vi "Clear Scan Time Out_2.vi"(6 "Channel number":i32, 7 "ESP32 ref":refnum<visa-resource-name>="COM4", 8 "error in (no error)":errorcluster, 11 "VISA Refnum in":refnum<visa-resource-name>) -> (0 "error out":errorcluster, 1 "error?":bool, 2 "Time out count":i32, 3 "VISA Refnum out":refnum<visa-resource-name>, 5 "ESP32 ref out":refnum<visa-resource-name>)   [LabVIEW 2023]
uses:
  <vilib>/Utility/error.llb/DialogType.ctl
panel:
  out "error out 3":errorcluster
  out "error out 2":errorcluster
  out "Measurements 3":dbl[](array[numeric])
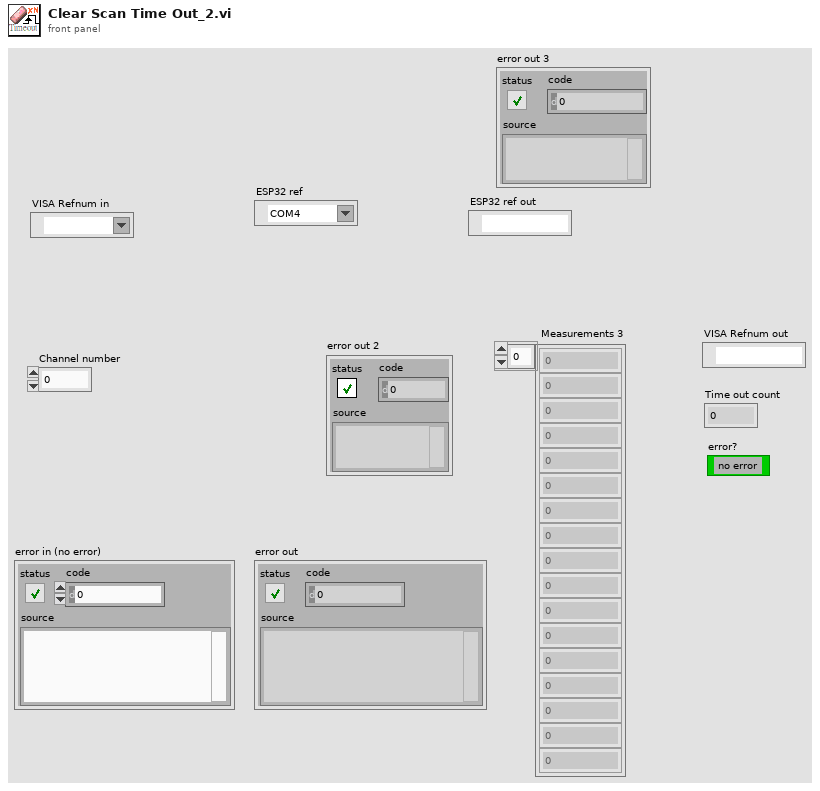
[diagram p1: front panel]
types:
  T1 = typedef "DialogType.ctl" = u16
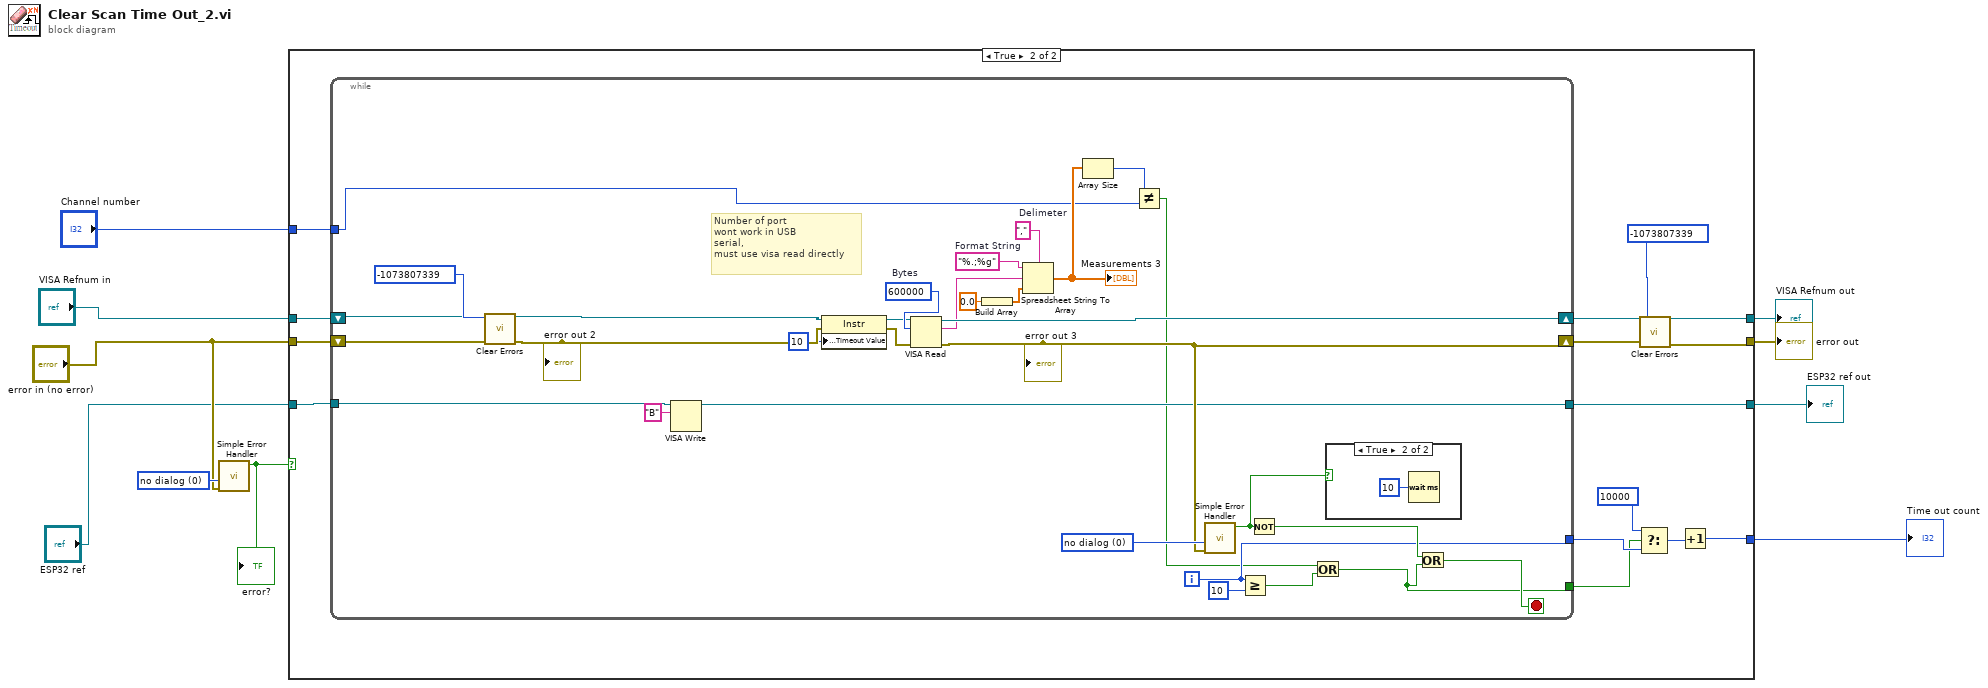
[diagram p0: block diagram]
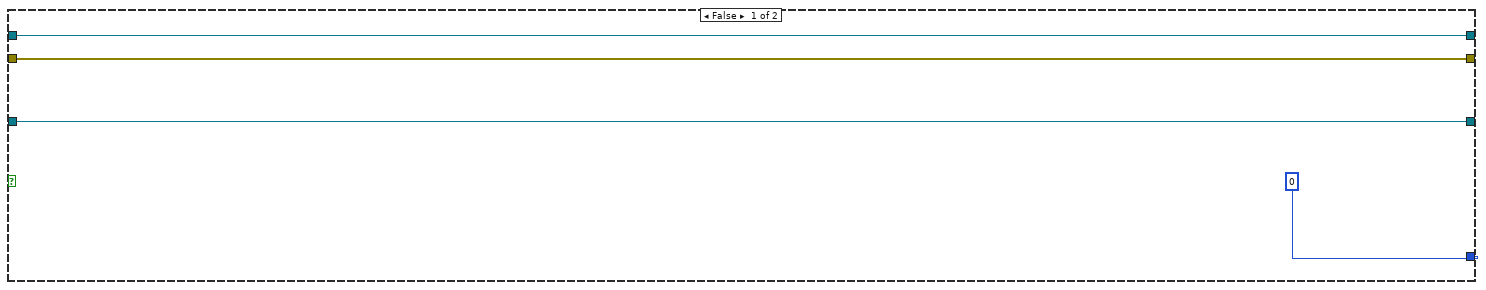
[diagram p2: hidden frame]
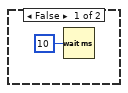
[diagram p3: hidden frame]
diagram:
  w7 = T1 0 items=["no dialog", "OK message", "continue or stop message", "OK message + warnings", "continue/stop + warnings"] ("type of dialog (OK msg:1)")
  n1 = call <vilib>:"Simple Error Handler.vi"("type of dialog (OK msg:1)"=w7, "error in (no error)"="error in (no error)") -> ("error?"=w5:bool)  [unwired: 3 in, 4 out]
  "error?" <- w5
  n2 = case shown="True" w5 {
    tunnel: [w14 w28] -> w10
    tunnel: "error in (no error)" -> [w13 w27]
    tunnel: "VISA Refnum in" -> [w14 w26]
    tunnel: [w13 w16] -> w8
    tunnel: [0 w25] -> w4
    tunnel: "ESP32 ref" -> [w11 w20]
    tunnel: [w11 w19] -> w2
    tunnel: "Channel number" -> [_ w18]
    frame False {
    }
    frame True {
      n3 = while {
        shift-right: [w53] -> w17
        shift-left: w27 -> [w56]
        shift-right: [w58] -> w28
        shift-left: w26 -> [w37]
        tunnel: [w49] -> w23
        tunnel: [w30] -> w22
        tunnel: w20 -> [w36]
        tunnel: [w35] -> w19
        tunnel: w18 -> [w32]
        i -> [w49]
        stop <- w50 stop-if-true
        w45 = ","  # Delimeter
        w46 = "%.;%g"  # Format String
        w41 = u32 600000  # Bytes
        w54 = T1 0 items=["no dialog", "OK message", "continue or stop message", "OK message + warnings", "continue/stop + warnings"] ("type of dialog (OK msg:1)")
        # "Number of port\nwont work in USB \nserial,\nmust use visa read directly"
        n4 = call <vilib>:"Clear Errors.vi"("error in (no error)"=w56, "specific error code to clear (0: all)"=-1073807339 ("code out")) -> ("error out"=w55:errorcluster)  [unwired: 4 in, 1 out]
        "error out 2" <- w55
        n5 = VISA Write(VISA resource name=w36, write buffer="B") -> (VISA resource name out=w35:refnum<visa-resource-name>)  [unwired: 1 in, 2 out]
        n6 = property class="Instr"(reference=w37, error in=w55, "General Settings:Timeout Value"=u32 10) -> (reference out=w40:refnum<visa-resource-name>, error out=w39:errorcluster)
        n7 = VISA Read(VISA resource name=w40, byte count=w41, error in (no error)=w39) -> (VISA resource name out=w58:refnum<visa-resource-name>, read buffer=w42:string, error out=w53:errorcluster)  [unwired: 1 out]
        "error out 3" <- w53
        n8 = Build Array(0.0) -> (w43:dbl[])
        n9 = Spreadsheet String To Array(delimiter (Tab)=w45, format string=w46, spreadsheet string=w42, array type (2D Dbl)=w43) -> (array=w34:dbl[])
        "Measurements 3" <- w34
        n10 = Array Size(array=w34) -> (size(s)=w33:i32)
        n11 = Not Equal?(x=w33, y=w32) -> (x != y?=w29:bool)
        n12 = call <vilib>:"Simple Error Handler.vi"("type of dialog (OK msg:1)"=w54, "error in (no error)"=w53) -> ("error?"=w48:bool)  [unwired: 3 in, 4 out]
        n13 = Greater Or Equal?(x=w49, y=10) -> (x >= y?=w31:bool)
        n14 = Not(x=w48) -> (.not. x?=w51:bool)
        n15 = Or(x=w29, y=w31) -> (x .or. y?=w30:bool)
        n16 = case shown="True" w48 {
          frame False {
            n17 = Wait (ms)(milliseconds to wait=u32 10) -> ()  [unwired: 1 out]
          }
          frame True {
            n18 = Wait (ms)(milliseconds to wait=u32 10) -> ()  [unwired: 1 out]
          }
        }
        n19 = Or(x=w51, y=w30) -> (x .or. y?=w50:bool)
      }
      n20 = Select(t=10000, s=w22, f=w23) -> (s? t:f=w24:i32)
      n21 = call <vilib>:"Clear Errors.vi"("error in (no error)"=w17, "specific error code to clear (0: all)"=-1073807339 ("code out")) -> ("error out"=w16:errorcluster)  [unwired: 4 in, 1 out]
      n22 = Increment(x=w24) -> (x+1=w25:i32)
    }
  }
  "error out" <- w8
  "VISA Refnum out" <- w10
  "Time out count" <- w4
  "ESP32 ref out" <- w2
